vi "Launch Autocomplete Handler.vi"(4 "Shared Options (Local)":refnum<class "Shared Options.lvclass">, 5 "Autohide ListBox (F)":bool, 6 "Allow Undefined Values (F)":bool, 7 "ListBox Refnum (Popup)":refnum<vi>, 8 "error in (no error)":errorcluster, 9 "Height (200)":i16=200, 10 "Initial Options (Empty)":string[](array[string]), 11 "Str Refnum":refnum<vi>) -> (0 "error out":errorcluster, 1 "New Options Event":refnum<user-event>, 2 "Stop Event":refnum<user-event>, 3 "Selection":refnum<user-event>)   [LabVIEW 2020, in "AutoComplete.lvlib"]
doc: "Creates a standalone AutoComplete handler with separate events for interaction. Register for the <b>Selection</b> event to receive selections made by users with autocomplete. <b>Stop</b> and <b>New Options</b> events are for interacting to the autocomplete handler.\n\n<b>Str Refnum</b> - The control that drives the search functionality and has the result placed in.\n<b>Initial Options</b> - The starting list of possible selections. This can bae updated later by generating a New Options event.\n<b>Height</b> - Sets the pixel height of the popup list when typing into the specified string.\n<b>ListBox Refnum</b> - Alternatively a separate ListBox can be specified that is integrated into the UI.\n<b>Autohide ListBox</b> - When specifying an external ListBox, this causes the listbox to be hidden whenever a selection is made.\n<b>Allow Undefined Values</b> - Allows users to enter arbitrary values in addition to what is available in the options list.\n<b>Shared Options</b> - Uses the Shared Options instance, if valid, to filter available options from. If a Shared Options instance is specified, the Selection event output will not be available for use."
uses:
  AutoComplete.lvlib
  Shared Options/Shared Options.lvclass
  Shared Options/Shared Options.lvclass/Shared Options.ctl
  Autocomplete UI.vi
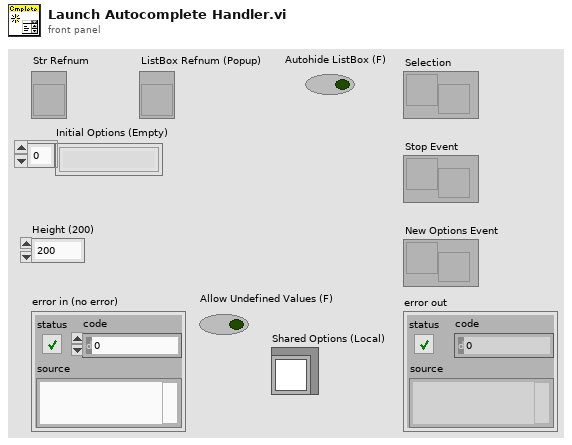
[diagram p1: front panel]
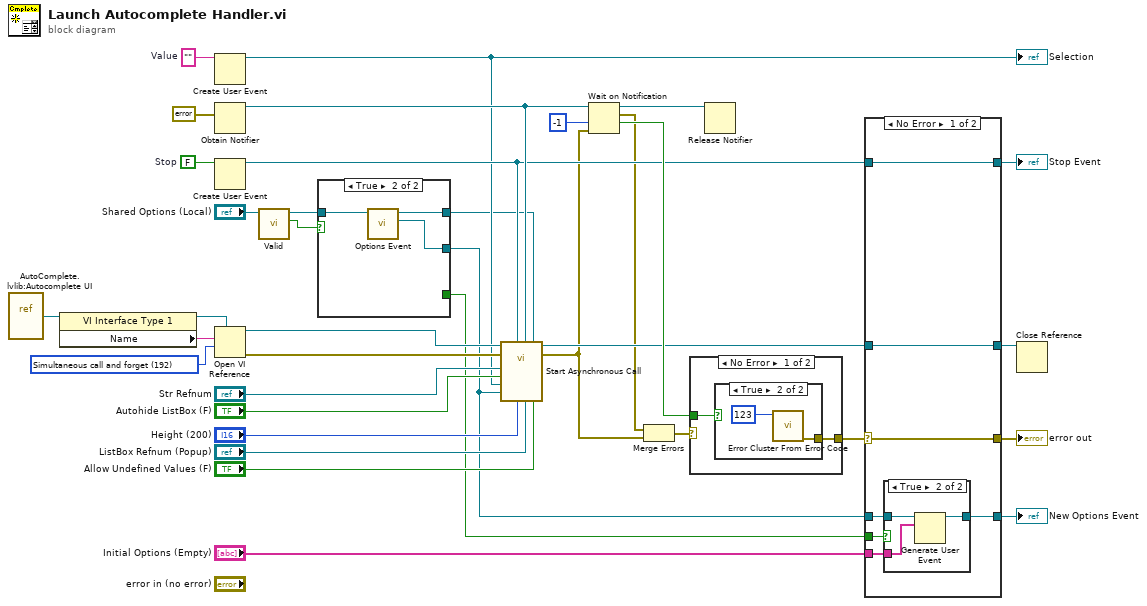
[diagram p0: block diagram]
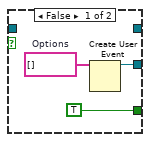
[diagram p2: hidden frame]
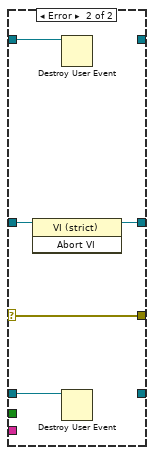
[diagram p6: hidden frame]
diagram:
  w9 = ""  # Value
  w32 = 192 items=["Record modifications"=1, "Open templates for editing"=2, "Prompt user to save"=4, "Prepare for reentrant run"=8, "Prompt to find missing subVIs"=16, "Hide loading dialog box"=32, "Enable simultaneous calls"=64, "Prepare to call and forget"=128, "Simultaneous call and forget"=192, "Prepare to call and collect"=256, "Simultaneous call and collect"=320]
  w36 = FALSE  # Stop
  n1 = vi-ref "AutoComplete.lvlib:Autocomplete UI.vi"() -> (w30:refnum<vi>)
  n2 = property class="VI Interface Type 1"(reference=w30) -> (reference out=w33:refnum<vi>, "Name"=w31:string)  [unwired: 1 in, 1 out]
  n3 = Create User Event(user event datatype=w9) -> (user event=w8:refnum<user-event>)  [unwired: 1 in, 1 out]
  "Selection" <- w8
  n4 = Obtain Notifier(notification data type=errorcluster {"status"=FALSE, "code"=0, "source"=""} ("error constant")) -> (notifier out=w26:refnum<notifier>)  [unwired: 3 in, 2 out]
  n5 = Create User Event(user event datatype=w36) -> (user event=w18:refnum<user-event>)  [unwired: 1 in, 1 out]
  n6 = Open VI Reference(type specifier VI Refnum (for type only)=w33, vi path=w31, options=w32) -> (vi reference=w35:refnum<vi>, error out=w34:errorcluster)  [unwired: 3 in]
  n7 = call "Valid.vi"("Shared Options in"="Shared Options (Local)") -> ("Valid"=w5:bool, "Shared Options out"=w4:refnum<class "Shared Options.lvclass">)  [unwired: 8 in, 1 out]
  n8 = case shown="True" w5 {
    tunnel: w4 -> [_ w42]
    tunnel: [w38 w40] -> w3
    tunnel: [_ w41] -> w2
    tunnel: [TRUE _] -> w1
    frame False {
      w39 = string[] []  # Options
      n9 = Create User Event(user event datatype=w39) -> (user event=w38:refnum<user-event>)  [unwired: 1 in, 1 out]
    }
    frame True {
      n10 = call "Options Event.vi"("Shared Options in"=w42) -> ("Options Event"=w40:refnum<user-event>, "Shared Options out"=w41:refnum<class "Shared Options.lvclass">)  [unwired: 8 in, 1 out]
    }
  }
  n11 = call-by-ref "Start Asynchronous Call"(reference=w35, error in=w34, "Allow Undefined Values? (F)"="Allow Undefined Values (F)", "Shared Options (Local)"=w2, "LstBox Refnum"="ListBox Refnum (Popup)", "Ready Notifier"=w26, "Height (200)"="Height (200)", "Stop Event"=w18, "Options"=w3, "Selection Event"=w8, "Autohide ListBox (F)"="Autohide ListBox (F)", "Str Refnum"="Str Refnum") -> (reference out=w21:refnum<vi>, error out=w12:errorcluster)  [unwired: 2 in]
  n12 = Wait on Notification(notifier=w26, timeout in ms (-1)=-1, error in (no error)=w12) -> (notifier out=w24:refnum<notifier>, notification=w14:errorcluster, timed out?=w23:bool)  [unwired: 1 in, 1 out]
  n13 = Merge Errors(w14, w12) -> (w13:errorcluster)
  n14 = case shown="No Error" w13 {
    selector: w13 -> [_ w47]
    tunnel: w23 -> [w44 _]
    tunnel: [w43 w47] -> w22
    frame No Error {
      n15 = case shown="True" w44 {
        tunnel: [_ w45] -> w43
        frame False {
        }
        frame True {
          n16 = call <vilib>:"Error Cluster From Error Code.vi"("error code (0)"=123) -> ("error out"=w45:errorcluster)  [unwired: 8 in]
        }
      }
    }
    frame Error {
    }
  }
  n17 = Release Notifier(notifier=w24) -> ()  [unwired: 2 in, 3 out]
  n18 = case shown="No Error" w22 {
    selector: w22 -> [w52 w58]
    tunnel: w3 -> [w51 w59]
    tunnel: w21 -> [w54 w62]
    tunnel: [w54 w61] -> w20
    tunnel: [w53 _] -> w19
    tunnel: w18 -> [w53 w60]
    tunnel: [w49 _] -> w17
    tunnel: [w52 w58] -> w16
    tunnel: "Initial Options (Empty)" -> [w50 _]
    tunnel: w1 -> [w48 _]
    frame No Error {
      n19 = case shown="True" w48 {
        tunnel: w51 -> [_ w57]
        tunnel: w50 -> [_ w56]
        tunnel: [_ w55] -> w49
        frame False {
        }
        frame True {
          n20 = Generate User Event(user event=w57, event data cluster=w56) -> (user event out=w55:refnum<user-event>)  [unwired: 2 in, 1 out]
        }
      }
    }
    frame Error {
      n21 = invoke class="VI (strict)" method="Abort VI"(reference=w62) -> (reference out=w61:refnum<vi>)  [unwired: 2 in, 2 out]
      n22 = Destroy User Event(user event=w60) -> ()  [unwired: 1 in, 1 out]
      n23 = Destroy User Event(user event=w59) -> ()  [unwired: 1 in, 1 out]
    }
  }
  "Stop Event" <- w19
  "New Options Event" <- w17
  "error out" <- w16
  n24 = Close Reference(reference=w20) -> ()  [unwired: 1 in, 1 out]
